vi "Actor Core.vi"(8 "error in":errorcluster, 11 "State in":refnum<class "Chef State.lvclass">) -> (0 "error out":errorcluster, 3 "Actor out":refnum<class "Actor.lvclass">)   [LabVIEW 2024, in "Chef States.lvlib" / "Chef State.lvclass"]
doc: "(<B>Filename</B>: Actor Framework.lvlib:Actor.lvclass:Actor Core.vi)\n\nThis override invokes Entry.vi on the initial state, prior to calling the parent Actor Core. Adding this behavior to Actor Core (instead of an override of Pre Launch Init.vi) allows the initial state to launch a nested actor as part of its entry behavior.\n\nReceives messages to the actor, reacts to them, and initiates any error handling that may shut the actor down.\n\nDescendant classes may override this VI to append parallel tasks for the actor to complete while it handles messages. Overrides use the Call Parent Method node."
uses:
  Chef State.lvclass
  <vilib>/ActorFramework/Actor/Actor.lvclass
  <vilib>/NI/Actors/State Actor/State Actor/State Actor.lvclass
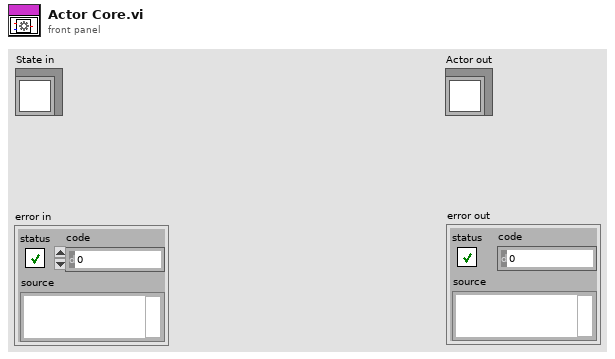
[diagram p1: front panel]
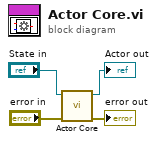
[diagram p0: block diagram]
diagram:
  n1 = call-parent "Actor Core.vi"("error in"="error in", "State in"="State in") -> ("error out"=→"error out":errorcluster, "Actor out"=→"Actor out":refnum<class "Actor.lvclass">)  [unwired: 8 in]
